vi "X3 solver.vi"(9 "q":dbl, 11 "p":dbl) -> (2 "X":dbl)   [LabVIEW 2014]
panel:
  # "Tartaglia-féle alak:X^3+pX+q=0"
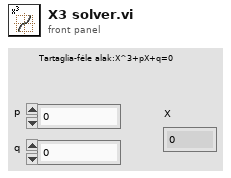
[diagram p1: front panel]
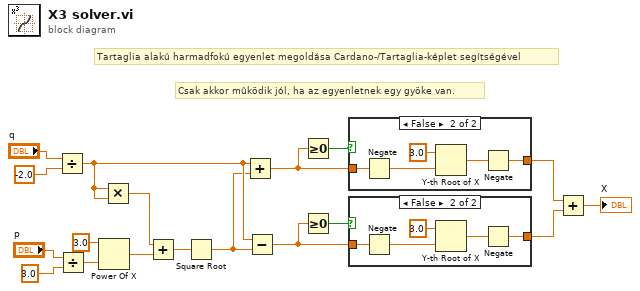
[diagram p0: block diagram]
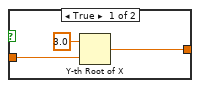
[diagram p2: hidden frame]
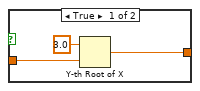
[diagram p3: hidden frame]
diagram:
  # "Csak akkor mûködik jól, ha az egyenletnek egy gyöke van."
  # "Tartaglia alakú harmadfokú egyenlet megoldása Cardano-/Tartaglia-képlet segítségével"
  n1 = Divide(x="q", y=-2.0) -> (x/y=w9:dbl)
  n2 = Divide(x="p", y=3.0) -> (x/y=w14:dbl)
  n3 = Power Of X(1:w14, 2:3.0 ("y")) -> (0:w11:dbl)
  n4 = Multiply(x=w9, y=w9) -> (x*y=w12:dbl)
  n5 = Add(x=w12, y=w11) -> (x+y=w10:dbl)
  n6 = Square Root(x=w10) -> (sqrt(x)=w8:dbl)
  n7 = Add(x=w9, y=w8) -> (x+y=w5:dbl)
  n8 = Subtract(x=w9, y=w8) -> (x-y=w3:dbl)
  n9 = Greater Or Equal To 0?(x=w5) -> (x >= 0?=w4:bool)
  n10 = Greater Or Equal To 0?(x=w3) -> (x >= 0?=w2:bool)
  n11 = case shown="False" w4 {
    tunnel: w5 -> [w21 w26]
    tunnel: [w19 w22] -> w7
    frame True {
      n12 = Y-th Root of X(1:w21, 2:3.0 ("y")) -> (0:w19:dbl)
    }
    frame False {
      n13 = Negate(x=w26) -> (-x=w23:dbl)
      n14 = Y-th Root of X(1:w23, 2:3.0 ("y")) -> (0:w24:dbl)
      n15 = Negate(x=w24) -> (-x=w22:dbl)
    }
  }
  n16 = case shown="False" w2 {
    tunnel: w3 -> [w29 w34]
    tunnel: [w27 w30] -> w1
    frame True {
      n17 = Y-th Root of X(1:w29, 2:3.0 ("y")) -> (0:w27:dbl)
    }
    frame False {
      n18 = Negate(x=w34) -> (-x=w31:dbl)
      n19 = Y-th Root of X(1:w31, 2:3.0 ("y")) -> (0:w32:dbl)
      n20 = Negate(x=w32) -> (-x=w30:dbl)
    }
  }
  n21 = Add(x=w7, y=w1) -> (x+y=→"X":dbl)
